vi "Draw Checkerboard.vi"(4 "CB type":u16, 5 "Resistance Read Ranges (2b)":dbl[](array[numeric]), 6 "CB size":i32, 7 "Resistance Read Ranges (1b)":dbl[](array[numeric]), 8 "error in (no error)":errorcluster, 9 "resistances (ohm)":dbl[][](array[numeric])) -> (0 "error out":errorcluster, 3 "Refnum out":T1)   [LabVIEW 2018]
uses:
  <vilib>/vision/Image Controls.llb/IMAQ Image.ctl
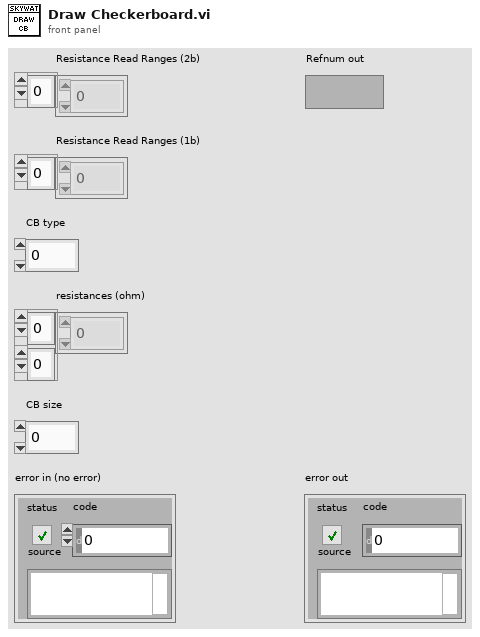
[diagram p1: front panel]
types:
  T1 = typedef "IMAQ Image.ctl" = refnum<image>
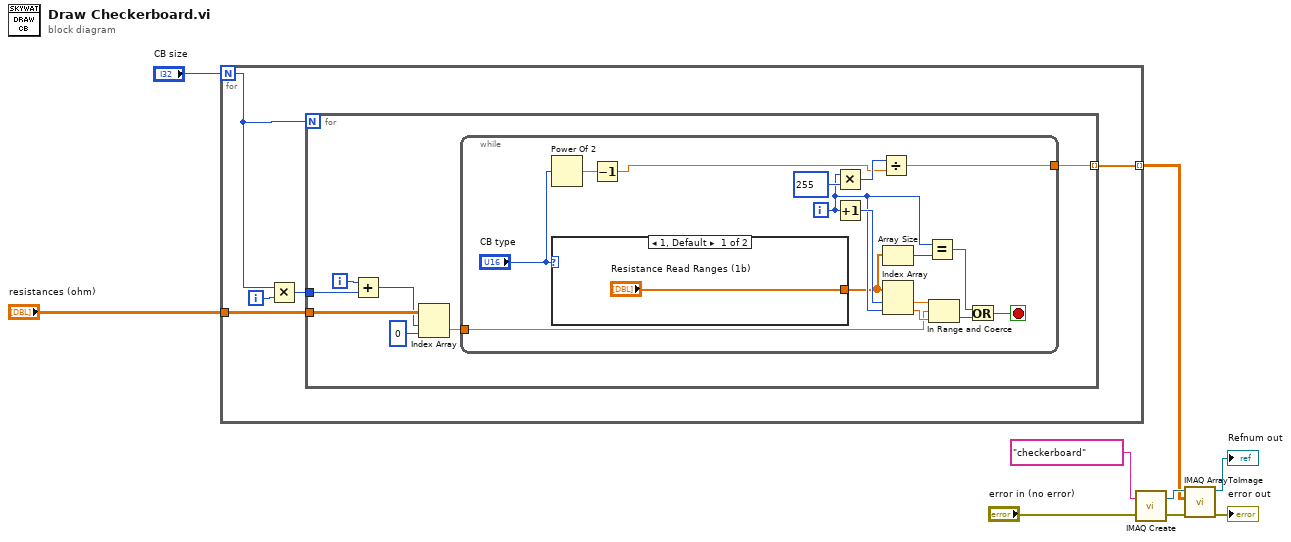
[diagram p0: block diagram]
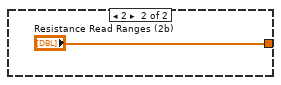
[diagram p2: hidden frame]
diagram:
  n1 = for {
    N: "CB size" -> [w12]
    tunnel: [w14] -> w5 mode=indexing
    tunnel: "resistances (ohm)" -> [w10]
    i -> [w13]
    n2 = Multiply(x=w12, y=w13) -> (x*y=w11:i32)
    n3 = for {
      N: w12 -> [_]
      tunnel: [w15] -> w14 mode=indexing
      tunnel: w11 -> [w20]
      tunnel: w10 -> [w19]
      i -> [w21]
      n4 = Add(x=w21, y=w20) -> (x+y=w17:i32)
      n5 = Index Array(array=w19, index (row)=w17, index (col)=0 ("disabled index (row)")) -> (element=w18:dbl)
      n6 = while {
        tunnel: [w28] -> w15
        tunnel: w18 -> [w34]
        i -> [w24]
        stop <- w27 stop-if-true
        n7 = Power Of 2(x="CB type") -> (2^x=w31:dbl)
        n8 = case shown="1, Default" "CB type" {
          tunnel: ["Resistance Read Ranges (1b)" "Resistance Read Ranges (2b)"] -> w22
          frame 1, Default {
          }
          frame 2 {
          }
        }
        n9 = Decrement(x=w31) -> (x-1=w29:dbl)
        n10 = Multiply(x=w24, y=255) -> (x*y=w32:i32)
        n11 = Increment(x=w24) -> (x+1=w37:i32)
        n12 = Divide(x=w32, y=w29) -> (x/y=w28:dbl)
        n13 = Array Size(array=w22) -> (size(s)=w23:i32)
        n14 = Index Array(array=w22, index #1=w37, index #2=w24) -> (element #1=w36:dbl, element #2=w35:dbl)
        n15 = Equal?(x=w24, y=w23) -> (x = y?=w25:bool)
        n16 = In Range and Coerce(upper limit=w36, x=w34, lower limit=w35) -> (In Range?=w26:bool)  [unwired: 1 out]
        n17 = Or(x=w25, y=w26) -> (x .or. y?=w27:bool)
      }
    }
  }
  n18 = call "IMAQ Create"("Image Name"="checkerboard", "error in (no error)"="error in (no error)") -> ("New Image"=w6:T1, "error out"=w4:errorcluster)  [unwired: 3 in]
  n19 = call "IMAQ ArrayToImage"("error in (no error)"=w4, "Image Pixels (U8)"=w5, "Image"=w6) -> ("error out"=→"error out":errorcluster, "Image Out"=→"Refnum out":T1)  [unwired: 7 in]
